vi "DTFT.vi"() -> ()   [LabVIEW 2014]
uses:
  <vilib>/Analysis/2dsp.llb/Real FFT.vi
  <vilib>/measure/NI_MAPro.lvlib
  <vilib>/Analysis/NI_AALPro.lvlib
panel:
  in  "signal type":T1(ring)
  in  "sampling info":cluster{"Fs":dbl, "#s":dbl}={"Fs"=1000.0, "#s"=1000.0} {"Fs" format="%.2p"}
  out "DTFT{x(n)}":cluster{"-pi to pi":dbl[], "DTFT op":dbl[]}(graph)
  out "graph of FFT":dbl[](graph)
  out "FFT {X}":cdb[](array[numeric])
  in  "Boolean":bool
  in  "formula":string="sin(w*t)*sin(2*pi(1)*t)"
  in  "Frequency":dbl(slide)=1.0 scale=0.0..500.0
  in  "Array":dbl[](array[numeric])
  out "ip waveform":dbl[](graph)
  in  "Select ip type":string(combo)
  out "Magnitude response":cluster{"-pi to pi":dbl[], "Magnitude op":dbl[]}(graph)
  out "|X(w)|":dbl[](array[numeric])
  out "X(w)":cdb[](array[numeric])
  # "Instructions"
  # "0<=freq<1/2(# of samples)"
  # "1. select the input type from drop down menu\n2. set the frequency desired with sampling info\n                        (or)\n     insert the formula with variable 't'\n                        (or)\n     insert values into array\n     (depending on the type of input)\n3. check the magnitude reponse with inbuilt function"
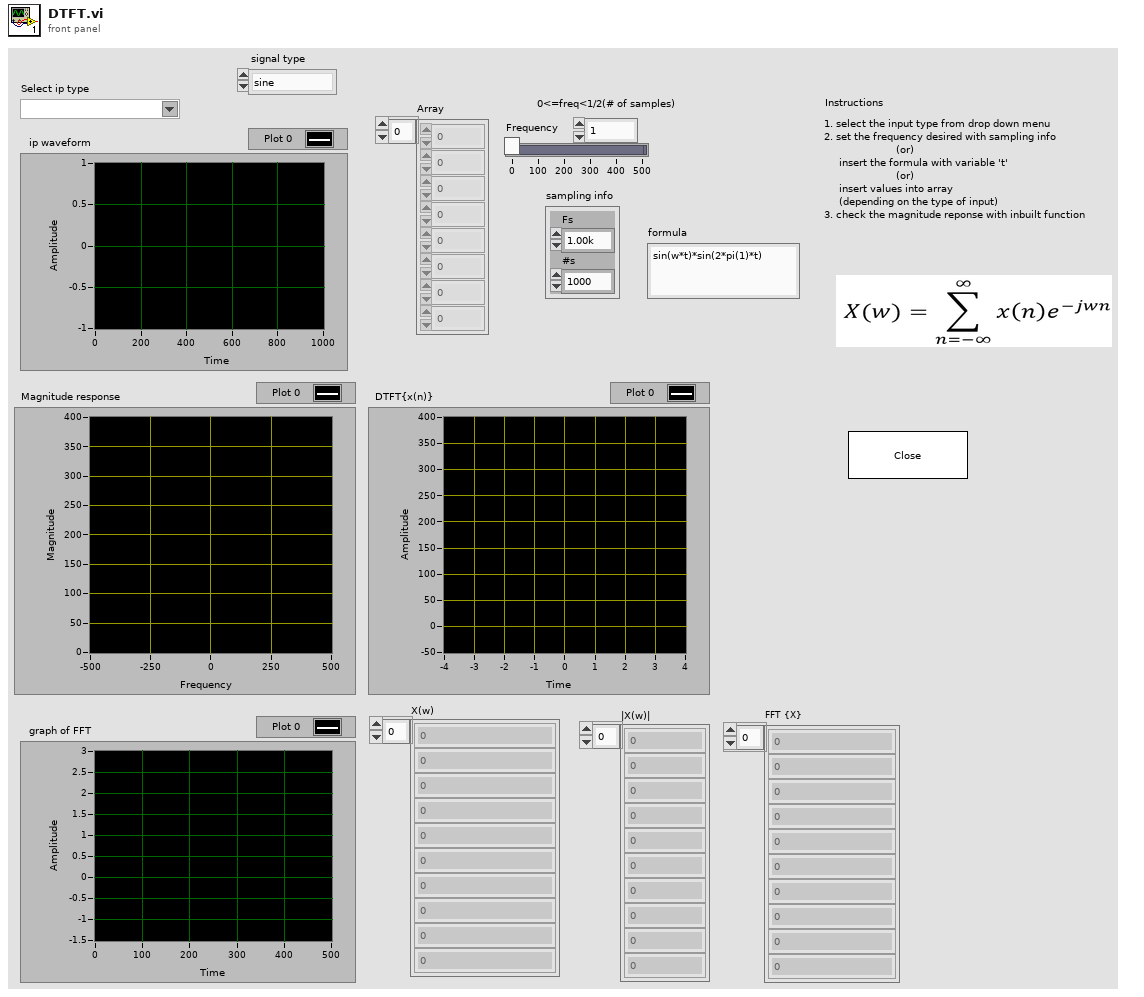
[diagram p1: front panel]
types:
  T1 = enum16{"sine", "cosine", "triangle", "square", "sawtooth", "increasing ramp", "decreasing ramp"}
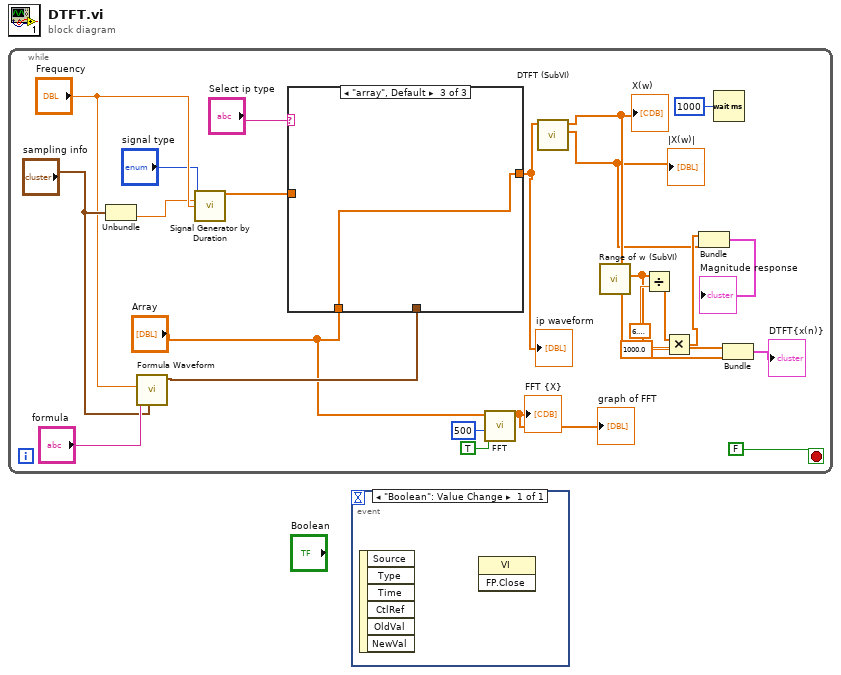
[diagram p0: block diagram]
diagram:
  n1 = while {
    stop <- FALSE ("stop") stop-if-true
    n2 = Unbundle("sampling info") -> ("#s"=w5:dbl)  [unwired: 1 out]
    n3 = call <vilib>:"Formula Waveform.vi"("sampling info"="sampling info", "formula"="formula", "amplitude"="Frequency") -> ("signal out"=w20:waveform(dbl))  [unwired: 7 in, 1 out]
    n4 = call <vilib>:"Signal Generator by Duration.vi"("signal type"="signal type", "# of samples"=w5, "frequency"="Frequency") -> ("signal"=w4:dbl[])  [unwired: 9 in, 3 out]
    n5 = case shown="\"array\", Default" "Select ip type" {
      tunnel: "Array" -> [_ _ w27]
      tunnel: w20 -> [_ w26 _]
      tunnel: w4 -> [w25 _ _]
      tunnel: [w25 w26 w27] -> w1
      frame "function generator" {
      }
      frame "formula" {
      }
      frame "array", Default {
      }
    }
    "ip waveform" <- w1
    n6 = call-poly <vilib>:"FFT.vi"("FFT size"=500, "shift?"=TRUE, "X"="Array") -> ("FFT {X}"=→"FFT {X}" →"graph of FFT":cdb[])  [unwired: 7 in, 1 out]
    n7 = call "DTFT (SubVI).vi"("ip array"=w1) -> ("Magnitude op"=w2:dbl[], "DTFT op"=w3:cdb[])  [unwired: 9 in]
    "X(w)" <- w3
    "|X(w)|" <- w2
    n8 = call "Range of w (SubVI).vi"() -> ("-pi to pi"=w11:dbl[])  [unwired: 11 in]
    n9 = Divide(x=w11, y=6.283185307179586) -> (x/y=w16:dbl[])
    n10 = Multiply(x=w16, y=1000.0) -> (x*y=w18:dbl[])
    n11 = Bundle(w18, "Magnitude op"=w2) -> (→"Magnitude response":cluster{dbl[], "Magnitude op":dbl[]})  [unwired: 1 in]
    n12 = Wait (ms)(milliseconds to wait=u32 1000) -> ()  [unwired: 1 out]
    n13 = Bundle("-pi to pi"=w11, "DTFT op"=w3) -> (→"DTFT{x(n)}":cluster{"-pi to pi":dbl[], "DTFT op":cdb[]})  [unwired: 1 in]
  }
  n14 = event shown="[0] \"Boolean\": Value Change" {
    selector: _ -> [_]
    dyn-events: _ -> [_]
    timeout: _ -> [_]
    event "Boolean": Value Change {
      n15 = event-data() -> ()  [unwired: 1 in, 6 out]
      n16 = invoke class="VI" method="FP.Close"() -> ()  [unwired: 3 in, 3 out]
    }
  }
